vi "stateMachine2.vi"() -> ()   [LabVIEW 2020]
uses:
  C:/Users/DESKTOP-TLO0G68A/Desktop/LabVIEW/instrumentationLV/Thorlabs.MotionControl.Controls.dll
  Thorlabs.MotionControl.Controls.dll
panel:
  in  "Numeric":i32
  in  "SerialNumber":string="27502753"
  in  "KCubeDCServoControl":refnum<k24>(container)
  in  "OK Button":bool
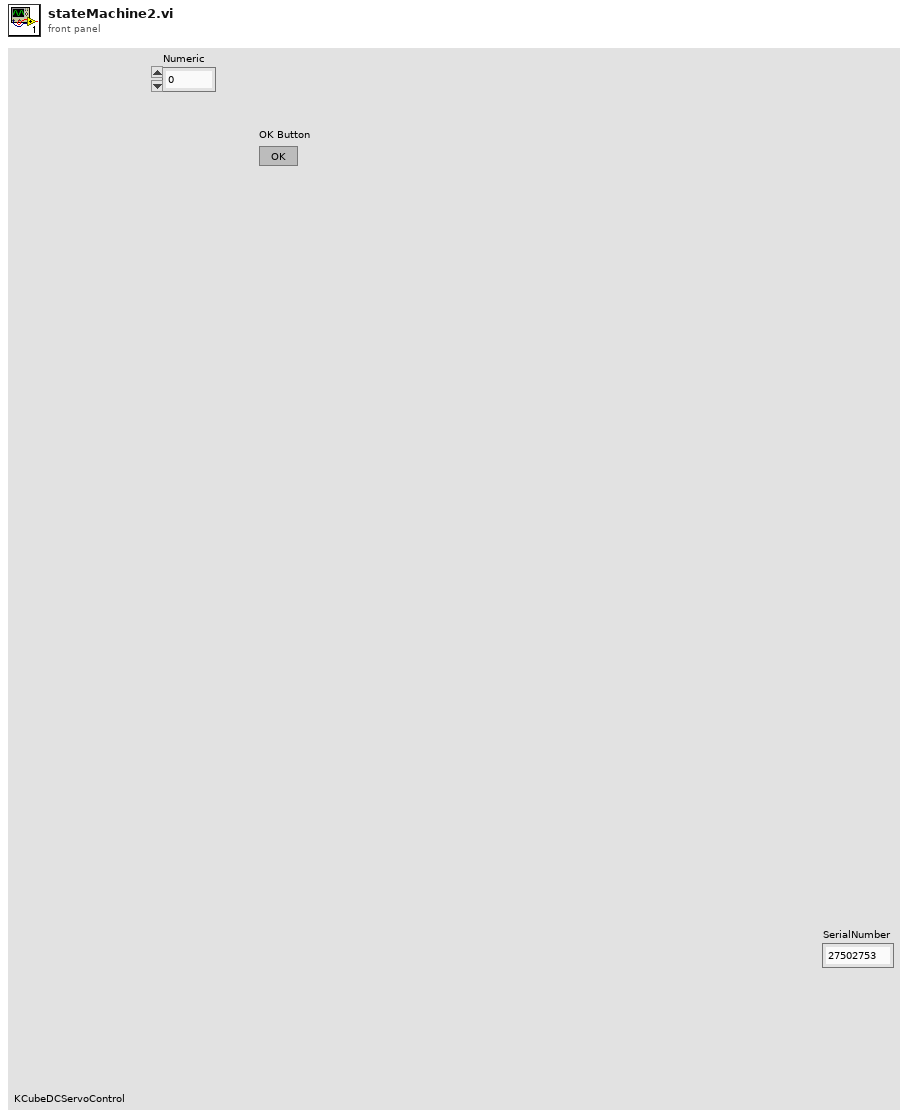
[diagram p1: front panel]
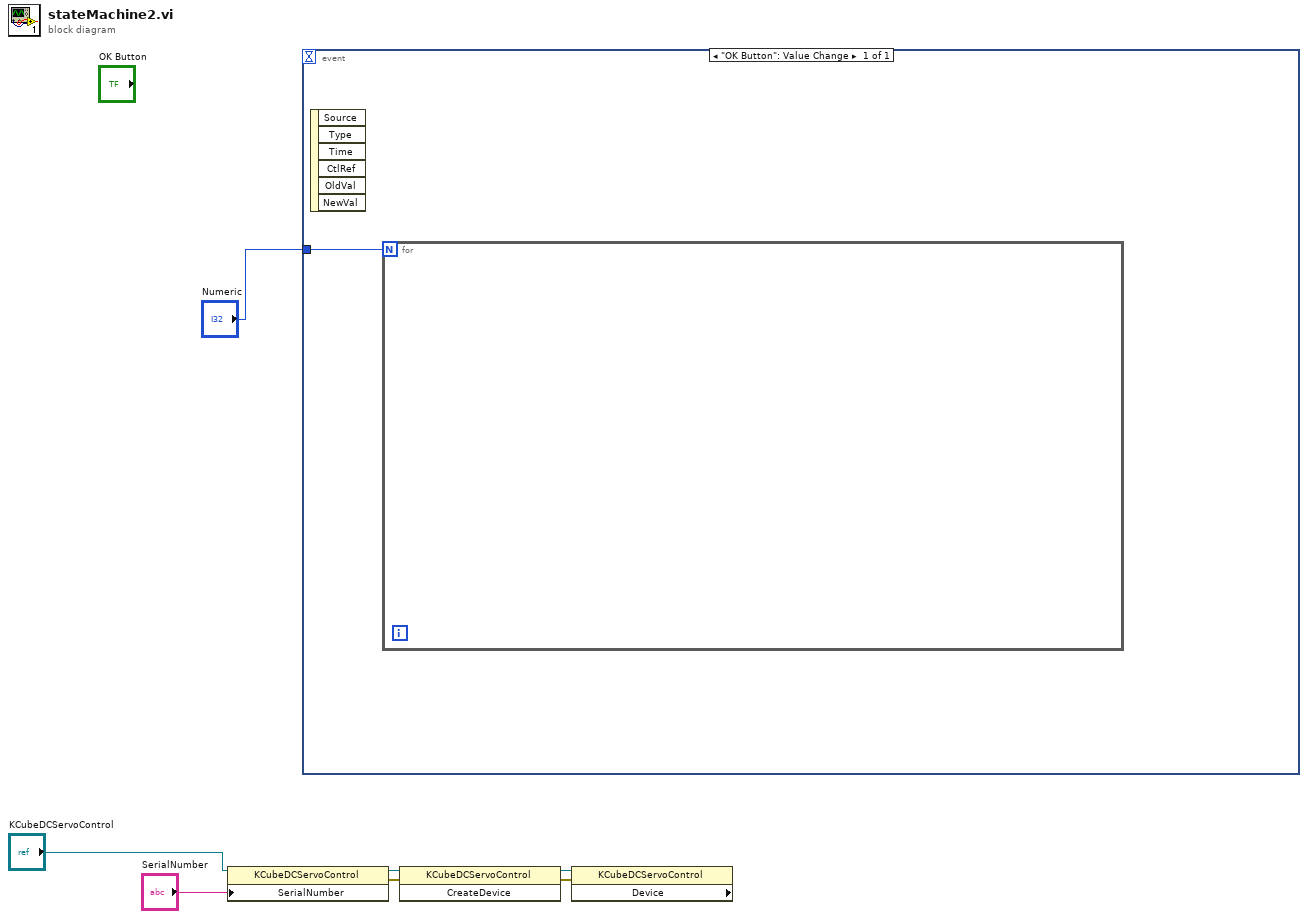
[diagram p0: block diagram]
diagram:
  n1 = property class="KCubeDCServoControl"(reference="KCubeDCServoControl", "SerialNumber"="SerialNumber") -> (reference out=w6:refnum<k24>, error out=w4:errorcluster)  [unwired: 1 in]
  n2 = event shown="[0] \"OK Button\": Value Change" {
    selector: _ -> [_]
    dyn-events: _ -> [_]
    timeout: _ -> [_]
    tunnel: "Numeric" -> [w8]
    event "OK Button": Value Change {
      n3 = event-data() -> ()  [unwired: 1 in, 6 out]
      n4 = for {
        N: w8 -> [_]
      }
    }
  }
  n5 = invoke class="KCubeDCServoControl" method="CreateDevice"(reference=w6, error in=w4) -> (reference out=w5:refnum<k24>, error out=w3:errorcluster)  [unwired: 1 in, 1 out]
  n6 = property class="KCubeDCServoControl" props=["Device"](reference=w5, error in=w3) -> ()  [unwired: 3 out]
